vi "Stop Core.vi"(10 "final error code":i32, 11 "Range Controller Actor in":refnum<class "Range Controller Actor.lvclass">) -> (3 "Range Controller Actor out":refnum<class "Range Controller Actor.lvclass">)   [LabVIEW 2018, in "Range Controller.lvlib" / "Range Controller Actor.lvclass"]
doc: "In addition to the following, this method also sends a message to the monitor to notify it that the actor has stopped execution.\n\n(<B>Filename</B>: Actor Framework.lvlib:Actor.lvclass:Stop Core.vi)\n\nDefines what the actor does before it stops. Use the <B>final error code</B> input to determine whether the actor shut down in response to an error.\n\nBy default, this method does nothing. A descendant class may override it to define behavior, such as shutting down any processes the actor initiated in its override of the Actor Core method.\n\nCopyright: MGI\nAuthored by: Derek Trepanier"
uses:
  Range Controller Actor.lvclass
  Range Controller Actor.lvclass/Range Controller Actor.ctl
  <vilib>/ActorFramework/Stop Msg/Stop Msg.lvclass/Stop Msg.ctl
  <vilib>/ActorFramework/Message Enqueuer/Message Enqueuer.lvclass/Message Enqueuer.ctl
  <vilib>/ActorFramework/Message Enqueuer/Enqueue Critical.vi
  <vilib>/ActorFramework/Stop Msg/Stop Msg.lvclass
  C:/Program Files (x86)/National Instruments/LabVIEW 2018/vi.lib/ActorFramework/Message/Message.lvclass
  <vilib>/ActorFramework/Message Priority Queue/Priority Enqueue.vi
  Actor Monitor/Actor/Monitored Actor.lvclass
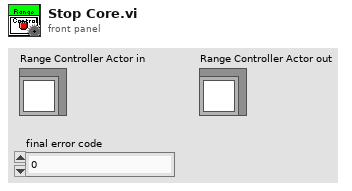
[diagram p1: front panel]
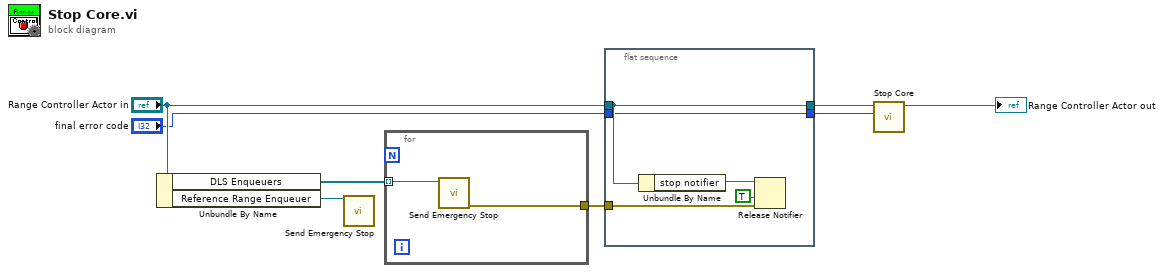
[diagram p0: block diagram]
diagram:
  n1 = Unbundle By Name("Range Controller Actor in") -> ("DLS Enqueuers"=w7:refnum<class "Message Enqueuer.lvclass">[], "Reference Range Enqueuer"=w4:refnum<class "Message Enqueuer.lvclass">)
  n2 = call <vilib>:"Send Emergency Stop.vi"("Message Enqueuer"=w4) -> ()  [unwired: 10 in, 1 out]
  n3 = for {
    tunnel: w7 -> [w10] mode=indexing
    tunnel: [w9] -> w5
    n4 = call <vilib>:"Send Emergency Stop.vi"("Message Enqueuer"=w10) -> ("error out"=w9:errorcluster)  [unwired: 10 in]
  }
  n5 = flat-sequence {
    tunnel: "Range Controller Actor in" -> [w12]
    tunnel: w5 -> [w13]
    tunnel: [w12] -> w3
    tunnel: "final error code" -> [w11]
    tunnel: [w11] -> w1
    frame #0 {
      n6 = Unbundle By Name(w12) -> ("stop notifier"=w15:refnum<notifier>)
      n7 = Release Notifier(notifier=w15, force destroy? (F)=TRUE, error in (no error)=w13) -> ()  [unwired: 3 out]
    }
  }
  n8 = call-parent "Stop Core.vi"("final error code"=w1, "Monitored Actor in"=w3) -> ("Monitored Actor out"=→"Range Controller Actor out":refnum<class "Range Controller Actor.lvclass">)  [unwired: 9 in]
